vi "XML_PASS_Iteme.vi"(0 "组合框":string(combo)="Double", 1 "Name":string, 2 "UpperLimit":string, 3 "Value":string, 4 "LowerLimit":string, 5 "MeasurementUnit":string, 6 "StatusCode":string) -> (20 "连接的字符串":string)   [LabVIEW 2018]
uses:
  Subvi/Global.vi
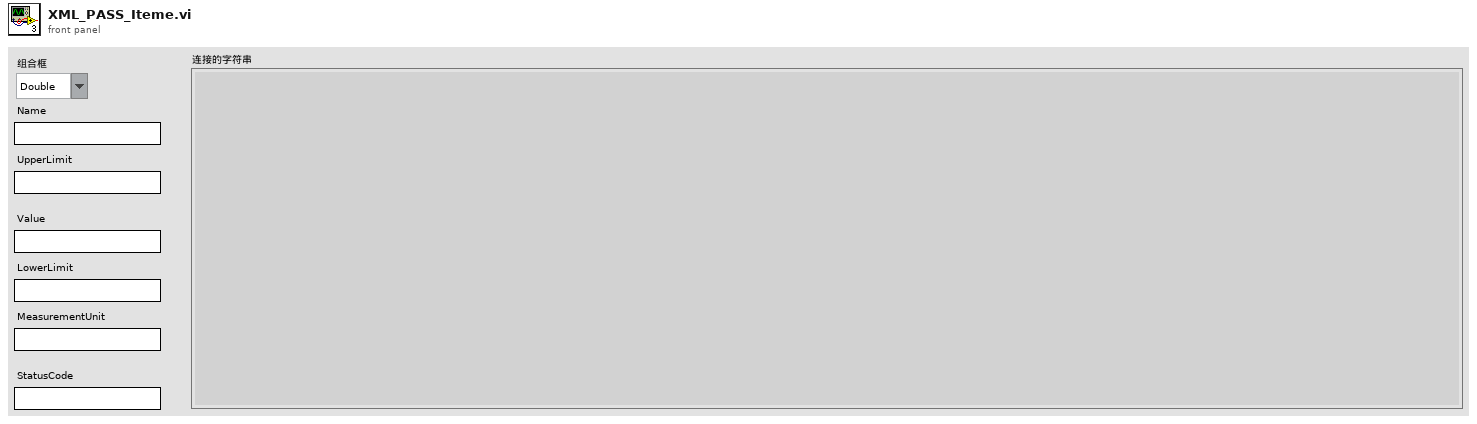
[diagram p1: front panel]
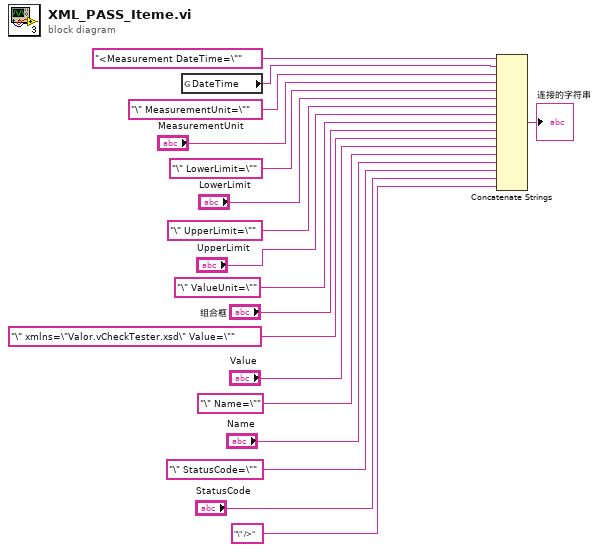
[diagram p0: block diagram]
diagram:
  n1 = global read "Global.vi" "DateTime"() -> (w17:string)
  n2 = Concatenate Strings("<Measurement DateTime=\"", w17, "\" MeasurementUnit=\"", "MeasurementUnit", "\" LowerLimit=\"", "LowerLimit", "\" UpperLimit=\"", "UpperLimit", "\" ValueUnit=\"", "组合框", "\" xmlns=\"Valor.vCheckTester.xsd\" Value=\"", "Value", "\" Name=\"", "Name", "\" StatusCode=\"", "StatusCode", "\" />") -> (→"连接的字符串":string)
